vi "Write All Elements Hidden.vi"(8 "error in (no error)":errorcluster, 10 "Correct. params. hidden":T1={"2nd image mirror axis"=1, "Cross-correlation decimation"=5, "Cross-correlation algorithm"=enum."frequency domain", "Always threshold when smoothing?"=TRUE, "Threshold only 2nd camera image?"=TRUE, "Median filter type"={"Order #"=4, "Y Size"=3, "X Size"=3}, "Gaussian filter kernel size"=3, "Gaussian filter kernel number"=3}, 11 "Correct params in":refnum<class "CV-Correction.lvclass">) -> (0 "error out":errorcluster, 3 "Correct params out":refnum<class "CV-Correction.lvclass">)   [LabVIEW 2013, in "CameraVision.lvlib" / "CV-Correction.lvclass"]
uses:
  CV-Correction.lvclass
  Correction-parameters-advanced.ctl
  CV-Correction.lvclass/CV-Correction.ctl
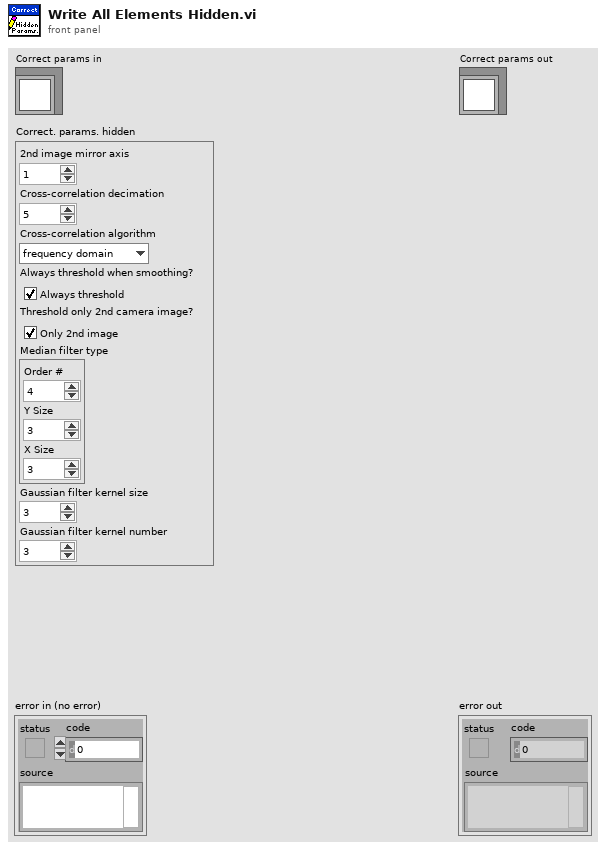
[diagram p1: front panel]
types:
  T1 = typedef "CameraVision.lvlib/CV-Correction.lvclass/Correction-parameters-advanced.ctl" = cluster{"2nd image mirror axis":u32, "Cross-correlation decimation":i32, "Cross-correlation algorithm":enum32{"direct", "frequency domain"}, "Always threshold when smoothing?":bool, "Threshold only 2nd camera image?":bool, "Median filter type":cluster{"Order #":i32, "Y Size":i32, "X Size":i32}, "Gaussian filter kernel size":i32, "Gaussian filter kernel number":i32}
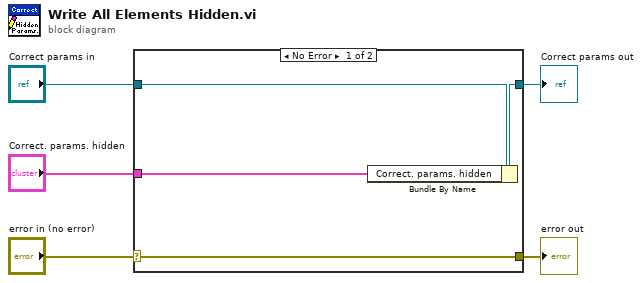
[diagram p0: block diagram]
diagram:
  n1 = case shown="No Error" "error in (no error)" {
    selector: "error in (no error)" -> [w9 w10]
    tunnel: [w9 w10] -> w4
    tunnel: [w7 w11] -> w2
    tunnel: "Correct params in" -> [w8 w11]
    tunnel: "Correct. params. hidden" -> [w6 _]
    frame No Error {
      n2 = Bundle By Name(cluster=w8, "Correct. params. hidden"=w6) -> (w7:refnum<class "CV-Correction.lvclass">)
    }
    frame Error {
    }
  }
  "error out" <- w4
  "Correct params out" <- w2
